vi "Add Client.vi"(8 "error in (no error)":errorcluster, 10 "Client":refnum<class "Websocket Client.lvclass">, 11 "Websocket Server in":refnum<class "Websocket Server.lvclass">) -> (0 "error out":errorcluster, 3 "Websocket Server out":refnum<class "Websocket Server.lvclass">)   [LabVIEW 2020, in "Stream-Websocket.lvlib" / "Websocket Server.lvclass"]
uses:
  Websocket Server.lvclass
  Websocket Server.lvclass/Websocket Server.ctl
  Server Connection Callback.vi
  Websocket Client/Websocket Client.lvclass
  C:/Program Files (x86)/National Instruments/LabVIEW 2020/vi.lib/IlluminatedG/lv-stream/Endpoint/Endpoint.lvclass
  C:/dev/IlluminatedG/lv-stream-websocket/Stream-Websocket/Websocket Server/Websocket Server.lvclass
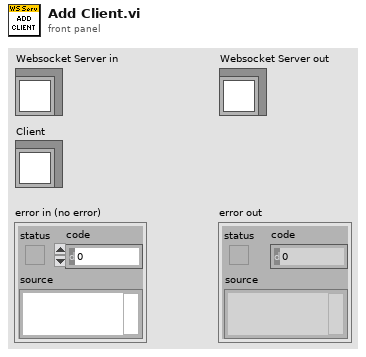
[diagram p1: front panel]
types:
  T1 = typedef "Stream-Websocket.lvlib/Websocket Server.lvclass/Ref Data.ctl" = cluster{"Listener":refnum<k5>, "Clients":refnum<class "Websocket Client.lvclass">[], "Server Loop":bool}
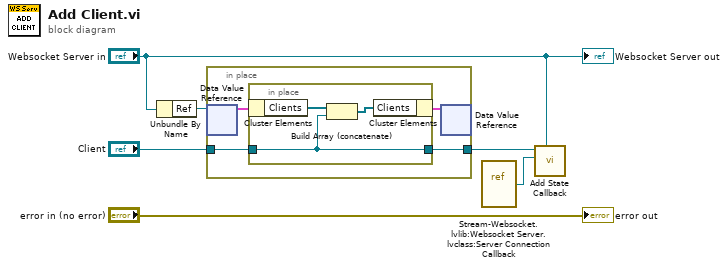
[diagram p0: block diagram]
diagram:
  n1 = Unbundle By Name("Websocket Server in") -> ("Ref"=w5:refnum<data-value>)
  n2 = in-place {
    in-place-border: "Client" -> [w8]
    in-place-border: [w7] -> w2
    n3 = in-place-dvr #1(w5) -> (w10:T1)  [unwired: 1 out]
    n4 = in-place {
      in-place-border: w8 -> [w11]
      in-place-border: [w11] -> w7
      n5 = in-place-cluster #2(w10) -> ("Clients"=w13:refnum<class "Websocket Client.lvclass">[])
      n6 = Build Array (concatenate)(w13, w11) -> (w12:refnum<class "Websocket Client.lvclass">[])
      n7 = in-place-cluster #2("Clients"=w12) -> (w9:T1)
    }
    n8 = in-place-dvr #1(w9) -> ()  [unwired: 2 out]
  }
  n9 = vi-ref "Stream-Websocket.lvlib:Websocket Server.lvclass:Server Connection Callback.vi"() -> (w1:refnum<vi>)
  n10 = call-dynamic "Add State Callback.vi"("Owner"="Websocket Server in", "Callback"=w1, "Connection in"=w2) -> ()  [unwired: 7 in, 2 out]
  "error out" <- "error in (no error)"
  "Websocket Server out" <- "Websocket Server in"
